vi "format floats for database.vi"(4 "Number":dbl) -> (1 "Insertion String":string)   [LabVIEW 2022 SP3, in "hse-db-ado.lvlib" / "ADO-DB-Driver.lvlib"]
doc: "Format float for database (either engineering format or NULL)\n\n____\nHAMPEL SOFTWARE ENGINEERING v1.4.0 (2023-12-19 09:52)"
uses:
  ADO-DB-Driver.lvlib
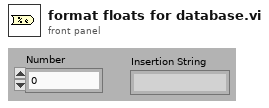
[diagram p1: front panel]
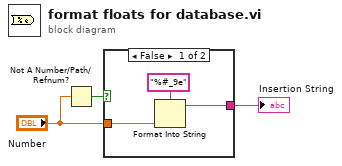
[diagram p0: block diagram]
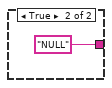
[diagram p2: hidden frame]
diagram:
  n1 = Not A Number/Path/Refnum?(number/path/refnum="Number") -> (NaN/Path/Refnum?=w3:bool)
  n2 = case shown="False" w3 {
    tunnel: "Number" -> [w5 _]
    tunnel: [w4 "NULL"] -> w2
    frame False {
      n3 = Format Into String(format string="%#_9e", w5) -> (resulting string=w4:string)  [unwired: 2 in, 1 out]
    }
    frame True {
    }
  }
  "Insertion String" <- w2
